vi "LuaVIEW Revoke Exports.vi"(5 "LuaVIEW reference in":T1, 11 "error in (no error)":errorcluster) -> (6 "LuaVIEW reference out":T1, 15 "error out":errorcluster)   [LabVIEW 2012]
doc: "Revokes the functions exported from a module or module instance. When your module performs cleanup actions after which calls to export functions result in erroneous or undefined results, and there is a risk that scripts that use the export functions are still active when your module cleans up, it is necessary to revoke the export functions before performing those cleanup actions. To do so, first call this VI from a dedicated module function, say \"revoke_exports()\". It is not fully safe to call this VI inside the cleanup function since an export call might be made in the short timespan between entering that function and revocation.\n\nNote that if you want the scripts that use the export functions to switch over to using a subsequently initialized module instance without their ongoing calls being in risk of failing, the new module instance must be initialized within the (configurable) \"export timeout\" period after this VI is called. This VI only throws an error when it is NOT called as part of a non-export module function."
uses:
  typedefs/t_LuaVIEW Reference.ctl
  typedefs/t_LuaVIEW CIN Spinlocked Actions.ctl
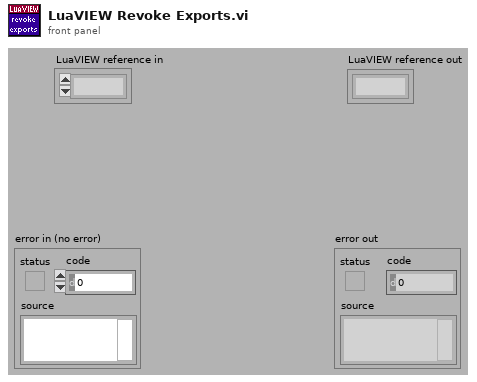
[diagram p1: front panel]
types:
  T1 = typedef "t_LuaVIEW Reference.ctl" = refnum<k1>
  T2 = typedef "t_LuaVIEW CIN Spinlocked Actions.ctl" = enum16{"totals", "taskcount", "open", "registerpublic", "registerexport", "revokeexports", "unregnextpublic", "usepublic", "pollexport", "close", "startyieldtest", "endyieldtest", "pollprintbuffer"}
  T3 = typedef "et_LuaVIEW CIN Results.ctl" = enum16{"OK", "error", "main", "call", "clonecall", "modulecall", "exportcall", "index", "yield"}
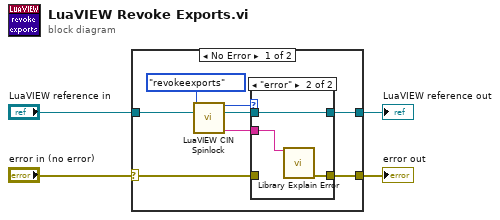
[diagram p0: block diagram]
diagram:
  n1 = case shown="No Error" "error in (no error)" {
    selector: "error in (no error)" -> [w6 w19]
    tunnel: [w8 w18] -> w4
    tunnel: [w5 w19] -> w3
    tunnel: "LuaVIEW reference in" -> [w12 w18]
    frame No Error {
      n2 = call "LuaVIEW CIN Spinlock.vi"("action"=t_LuaVIEW_CIN_Spinlocked_Actions."revokeexports", "LuaVIEW reference in"=w12) -> ("result"=w10:T3, "LuaVIEW reference out"=w9:T1, "string out"=w7:string)  [unwired: 7 in, 4 out]
      n3 = case shown="\"error\"" w10 {
        tunnel: w9 -> [w13 w17]
        tunnel: [w13 w17] -> w8
        tunnel: w7 -> [_ w16]
        tunnel: [w14 w15] -> w5
        tunnel: w6 -> [w14 _]
        frame Default {
        }
        frame "error" {
          n4 = call "Library Explain Error.vi"("explanation prefix (none)"=w16) -> ("explained error"=w15:errorcluster)  [unwired: 14 in]
        }
      }
    }
    frame Error {
    }
  }
  "LuaVIEW reference out" <- w4
  "error out" <- w3
